vi "Oxford visa write read.vi"(8 "error in (no error)":errorcluster, 9 "milliseconds to wait":u32, 10 "write buffer":string, 11 "VISA resource name":refnum<visa-resource-name>) -> (0 "error out":errorcluster, 2 "read buffer":string, 3 "VISA resource name out":refnum<visa-resource-name>)   [LabVIEW 2016]
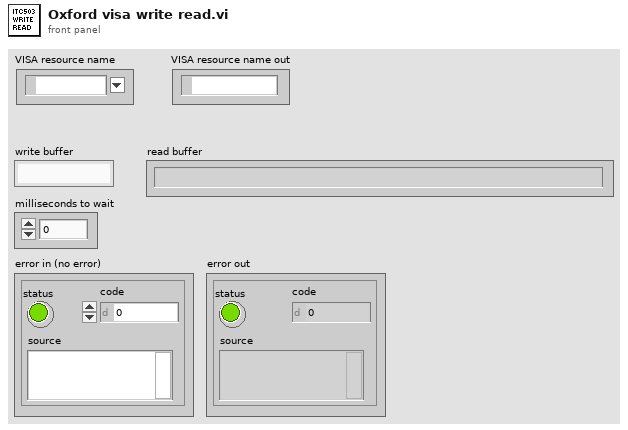
[diagram p1: front panel]
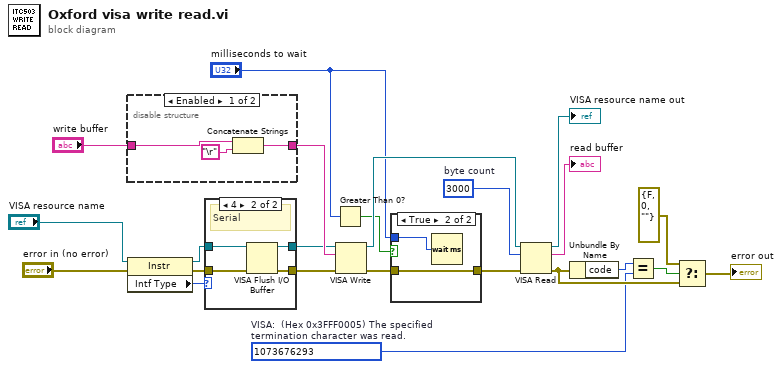
[diagram p0: block diagram]
diagram:
  w19 = 1073676293  # VISA:  (Hex 0x3FFF0005) The specified termination character was read.
  w16 = u32 3000  # byte count
  n1 = disable-structure shown="Enabled" {
    disable-tunnel: "write buffer" -> [w26 w27]
    disable-tunnel: [w25 w27] -> w12
    frame Enabled {
      n2 = Concatenate Strings(w26, "\r") -> (w25:string)
    }
    frame Disabled {
    }
  }
  n3 = property class="Instr"(reference="VISA resource name", error in="error in (no error)") -> (reference out=w6:refnum<visa-resource-name>, error out=w5:errorcluster, "Intf Type"=w7:u16)
  n4 = case shown="4" w7 {
    tunnel: w5 -> [w28 w33]
    tunnel: [w28 w32] -> w1
    tunnel: [w29 w31] -> w2
    tunnel: w6 -> [w29 w30]
    frame 0, Default {
    }
    frame 4 {
      # "Serial"
      n5 = VISA Flush I/O Buffer(VISA resource name=w30, error in (no error)=w33) -> (VISA resource name out=w31:refnum<visa-resource-name>, error out=w32:errorcluster)  [unwired: 1 in]
    }
  }
  n6 = Greater Than 0?(x="milliseconds to wait") -> (x > 0?=w11:bool)
  n7 = VISA Write(VISA resource name=w2, write buffer=w12, error in (no error)=w1) -> (VISA resource name out=w15:refnum<visa-resource-name>, error out=w9:errorcluster)  [unwired: 1 out]
  n8 = case shown="True" w11 {
    tunnel: "milliseconds to wait" -> [_ w36]
    tunnel: w9 -> [w34 w35]
    tunnel: [w34 w35] -> w8
    frame False {
    }
    frame True {
      n9 = Wait (ms)(milliseconds to wait=w36) -> ()  [unwired: 1 out]
    }
  }
  n10 = VISA Read(VISA resource name=w15, byte count=w16, error in (no error)=w8) -> (VISA resource name out=→"VISA resource name out":refnum<visa-resource-name>, read buffer=→"read buffer":string, error out=w21:errorcluster)  [unwired: 1 out]
  n11 = Unbundle By Name(w21) -> ("code"=w18:i32)
  n12 = Equal?(x=w18, y=w19) -> (x = y?=w22:bool)
  n13 = Select(t=errorcluster {"status"=FALSE, "code"=0, "source"=""}, s=w22, f=w21) -> (s? t:f=→"error out":errorcluster)
